vi "4.6.2.vi"() -> ()   [LabVIEW 2017]
panel:
  in  "停止":bool
  out "和":dbl
  in  "加数 2":dbl
  in  "加数1":dbl
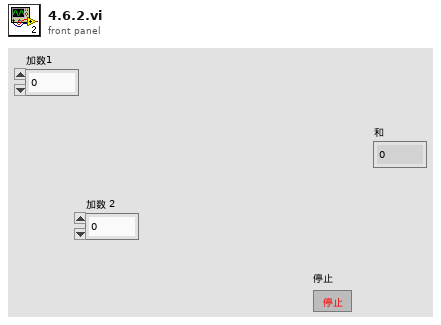
[diagram p1: front panel]
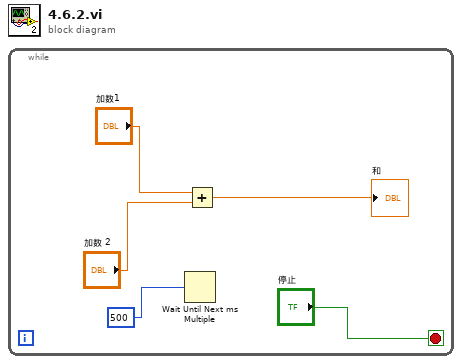
[diagram p0: block diagram]
diagram:
  n1 = while {
    stop <- "停止" stop-if-true
    n2 = Wait Until Next ms Multiple(millisecond multiple=500) -> ()  [unwired: 1 out]
    n3 = Add(x="加数1", y="加数 2") -> (x+y=→"和":dbl)
  }
